vi "Position yes no Cancel Button.vi"(8 "error in (no error)":errorcluster, 10 "Message":refnum<vi>, 11 "Button Ref":refnum<vi>) -> (0 "error out":errorcluster)   [LabVIEW 2014]
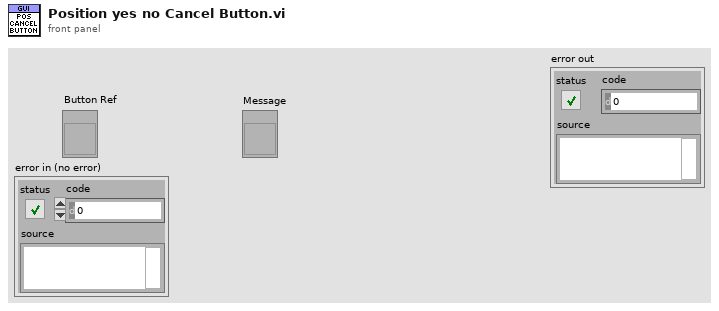
[diagram p1: front panel]
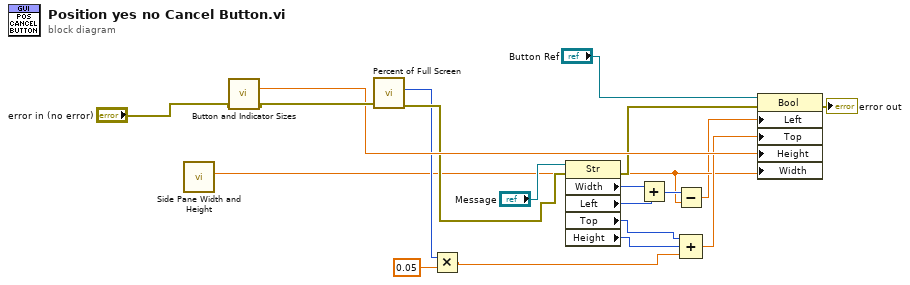
[diagram p0: block diagram]
diagram:
  n1 = call "Side Pane Width and Height.vi"() -> ("Width"=w2:dbl)  [unwired: 9 in, 2 out]
  n2 = call "Button and Indicator Sizes.vi"("error in (no error)"="error in (no error)") -> ("Button Height"=w15:dbl, "error out"=w17:errorcluster)  [unwired: 10 in, 3 out]
  n3 = call "Percent of Full Screen.vi"("error in (no error)"=w17) -> ("error out"=w13:errorcluster, "Bottom"=w8:i16)  [unwired: 8 in, 1 out]
  n4 = Multiply(x=w8, y=0.05) -> (x*y=w6:dbl)
  n5 = property class="Str"(reference="Message", error in=w13) -> (error out=w12:errorcluster, "Width"=w5:u32, "Left"=w4:i32, "Top"=w11:i32, "Height"=w10:u32)  [unwired: 1 out]
  n6 = Add(x=w5, y=w4) -> (x+y=w3:u32)
  n7 = Subtract(x=w3, y=w2) -> (x-y=w1:dbl)
  n8 = Compound Arithmetic op=ADD(w11, w10, w6) -> (w9:dbl)
  n9 = property class="Bool"(reference="Button Ref", error in=w12, "Left"=w1, "Top"=w9, "Height"=w15, "Width"=w2) -> (error out=→"error out":errorcluster)  [unwired: 1 out]
